vi "06 Shift Registers.vi"() -> ()   [LabVIEW 2020]
uses:
  _Subs/OpenDiagram/Open_XControl.xctl
panel:
  in  "OpenDiag":refnum<vi>(xcontrol)
  out "n!":i32=120
  in  "n":i32=5
  # "06 Shift Registers\nThis code demonstrates how shift registers work\n\nInstructions:\n1. Select Highlight Execution (light bulb on diagram)\n2. Hit run and watch the values on the wires change"
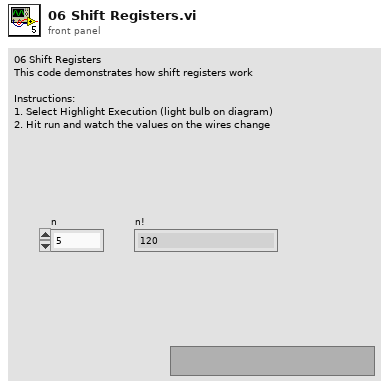
[diagram p1: front panel]
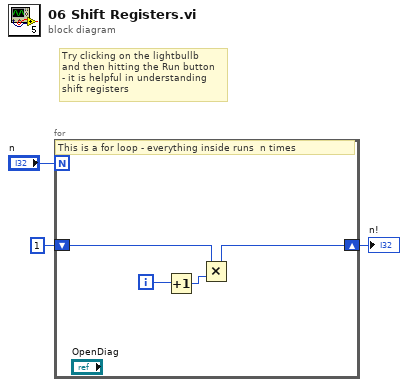
[diagram p0: block diagram]
diagram:
  # "Try clicking on the lightbullb\nand then hitting the Run button\n- it is helpful in understanding \nshift registers"
  n1 = for {
    N: "n" -> [_]
    shift-right: [w4] -> w1
    shift-left: 1 -> [w5]
    i -> [w7]
    # "This is a for loop - everything inside runs  n times"
    n2 = Increment(x=w7) -> (x+1=w6:i32)
    n3 = Multiply(x=w5, y=w6) -> (x*y=w4:i32)
  }
  "n!" <- w1
